vi "Boiler room.vi"() -> ()   [LabVIEW 2023]
panel:
  in  "Automatic / Manual":bool
  in  "max temp":dbl=80.0
  in  "min temp":dbl=20.0
  in  "stop":bool
  out "AC":bool
  out "Heater":bool
  out "Manual":bool
  in  "Heater":bool
  in  "AC":bool
  in  "Thermometer":dbl(slide) scale=0.0..100.0
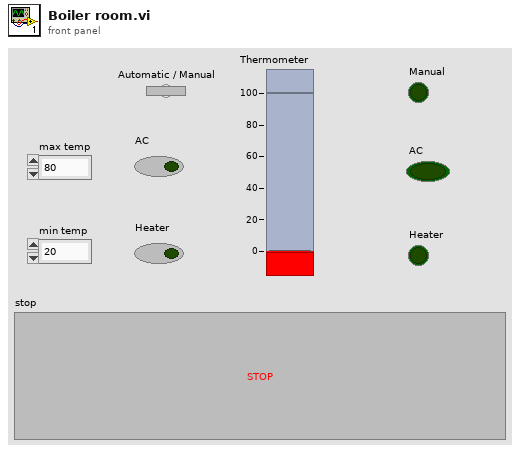
[diagram p1: front panel]
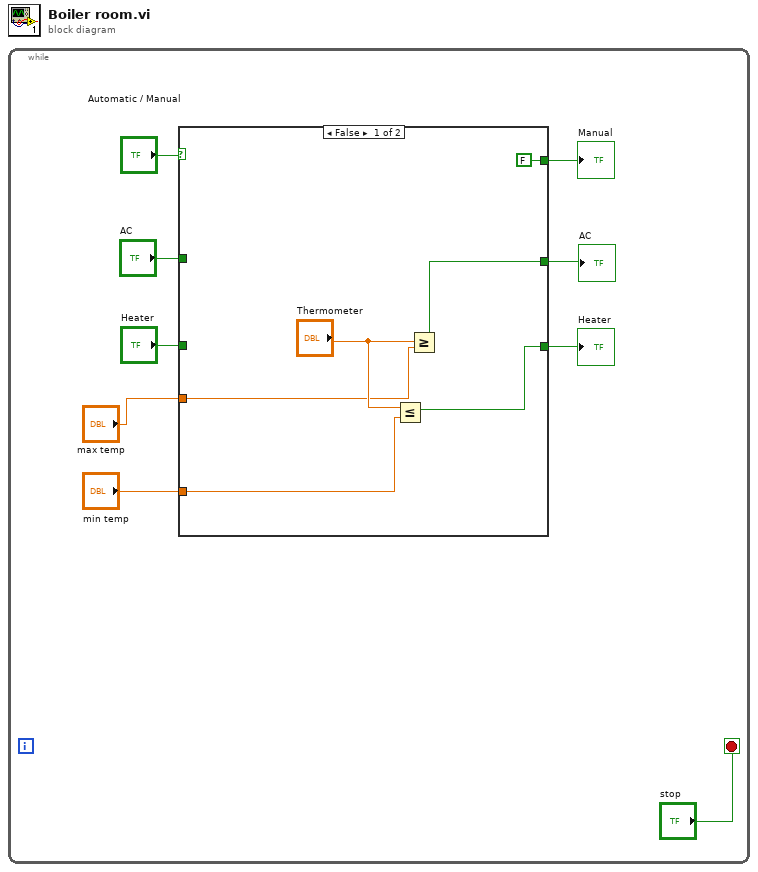
[diagram p0: block diagram]
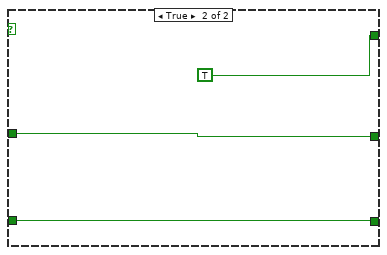
[diagram p2: hidden frame]
diagram:
  n1 = while {
    stop <- "stop" stop-if-true
    n2 = case shown="False" "Automatic / Manual" {
      tunnel: [w14 w18] -> w3
      tunnel: "Heater" -> [_ w18]
      tunnel: [w15 w17] -> w7
      tunnel: "AC" -> [_ w17]
      tunnel: [FALSE TRUE] -> w6
      tunnel: "max temp" -> [w11 _]
      tunnel: "min temp" -> [w10 _]
      frame False {
        n3 = Less Or Equal?(x="Thermometer", y=w10) -> (x <= y?=w14:bool)
        n4 = Greater Or Equal?(x="Thermometer", y=w11) -> (x >= y?=w15:bool)
      }
      frame True {
      }
    }
    "Manual" <- w6
    "Heater" <- w3
    "AC" <- w7
  }
